vi "32.vi"(9 "3":dbl, 10 "Numeric":i32, 11 "Numeric 2":i32) -> (3 "Array":u32[](array[numeric]))   [LabVIEW 2016]
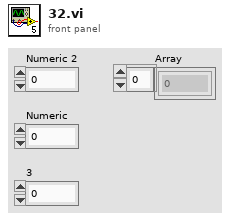
[diagram p1: front panel]
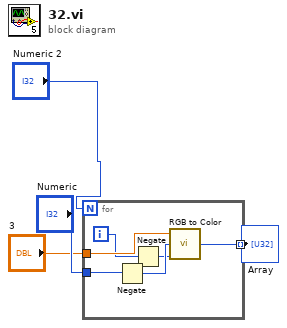
[diagram p0: block diagram]
diagram:
  n1 = for {
    N: "Numeric 2" -> [_]
    tunnel: [w10] -> w4 mode=indexing
    tunnel: "3" -> [w9]
    tunnel: "Numeric" -> [w8]
    i -> [w5]
    n2 = Negate(x=w8) -> (-x=w7:i32)
    n3 = Negate(x=w5) -> (-x=w6:i32)
    n4 = call <vilib>:"RGB to Color.vi"("B"=w6, "G"=w7, "R"=w9) -> ("Color"=w10:u32)
  }
  "Array" <- w4
